vi "ReadMNValuesJSON_EditTolerance_MultipleRacks.vi"(8 "error in":errorcluster, 11 "JSON file path":path=path "C:/Users/raakeshs/Desktop/ppts/JSON/Write to JSON String/data/Files/test4.json") -> (0 "error out":errorcluster, 3 "Rack Controller Parameters out":T1)   [LabVIEW 2015, in "ZenGage v3.0 UI.lvclass"]
uses:
  ZenGage v3.0 UI.lvclass
panel:
  out "VCluster\n out":variant
  out "Error Message":string
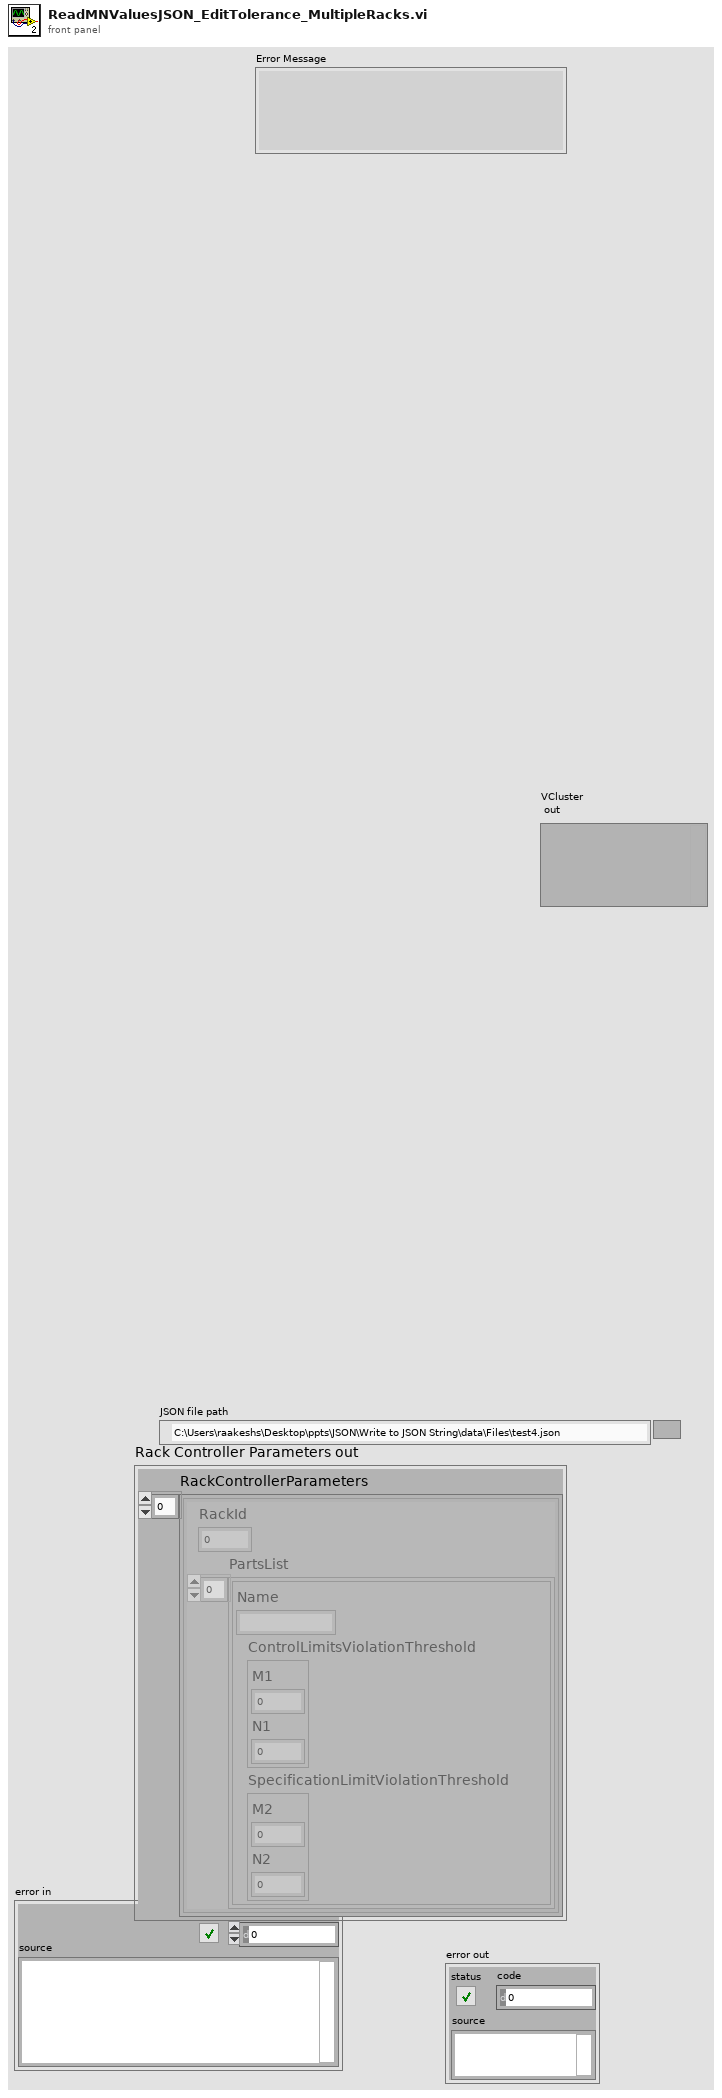
[diagram p1: front panel]
types:
  T1 = cluster{"RackControllerParameters":cluster{"RackId":i32, "PartsList":cluster{"Name":string, "ControlLimitsViolationThreshold":cluster{"M1":u64, "N1":u64}, "SpecificationLimitViolationThreshold":cluster{"M2":u64, "N2":u64}}[]}[]}
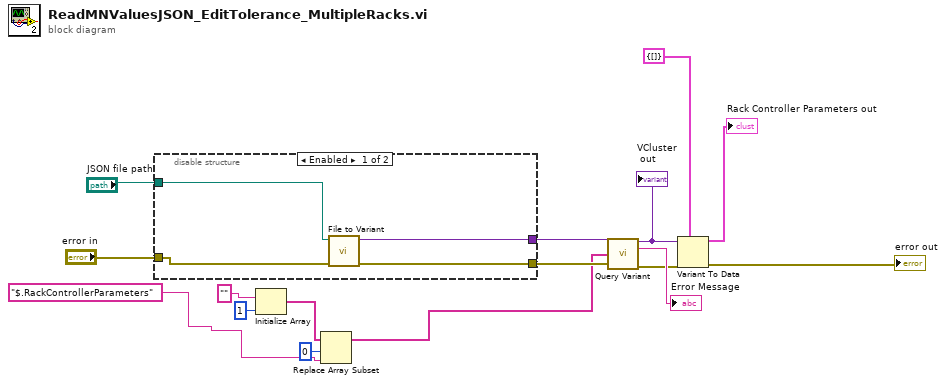
[diagram p0: block diagram]
diagram:
  n1 = disable-structure shown="Enabled" {
    disable-tunnel: [w19 w21] -> w16
    disable-tunnel: "error in" -> [w20 w21]
    disable-tunnel: "JSON file path" -> [w18 _]
    disable-tunnel: [w17 _] -> w1
    frame Enabled {
      n2 = call <vilib>:"File to Variant.vi"("JSON FilePath"=w18, "error in (no error)"=w20) -> ("JSON Variant"=w17:variant, "error out"=w19:errorcluster)  [unwired: 6 in, 1 out]
    }
    frame Disabled {
    }
  }
  n3 = Initialize Array("", 1 ("dimension size")) -> (w9:string[])
  n4 = Replace Array Subset(array=w9, new element="$.RackControllerParameters" ("string"), index=0) -> (w8:string[])
  n5 = call <vilib>:"Query Variant.vi"("VCluster in"=w1, "pathList"=w8, "error IO"=w16) -> ("VCluster\n out"=w14:variant, "Error Message"=→"Error Message":string, "error out"=w12:errorcluster)  [unwired: 9 in, 1 out]
  "VCluster\n out" <- w14
  n6 = Variant To Data(error in=w12, type=T1 {"RackControllerParameters"=[]}, Variant=w14) -> (data=→"Rack Controller Parameters out":T1, error out=→"error out":errorcluster)
